vi "4080_Comms.vi"(4 "Value to display":dbl min=0.0 max=9999.9 format="%.1f", 5 "Function":T2, 6 "Channel Name":string, 9 "Address":T1) -> (1 "Reading":dbl, 2 "millisecond timer value":u32, 3 "Comment":string)   [LabVIEW 2018]
uses:
  ADAM Client/Sub VIs/ADAM Controls/Function_ADAM.ctl
  ADAM Client/Sub VIs/ADAM Controls/Address.ctl
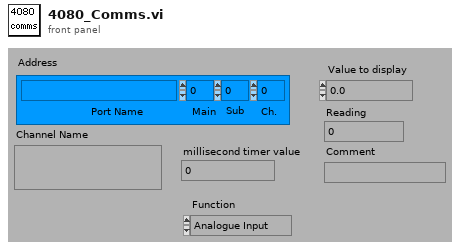
[diagram p1: front panel]
types:
  T1 = typedef "Address.ctl" = cluster{"Main":i32, "Ch.":i32, "Sub":i32, "Port Name":string}
  T2 = typedef "Function_ADAM.ctl" = enum16{"Analogue Input", "Digital Input", "Event counter", "Event rate", "Analogue Output", "Digital Output", "Relay Output"}
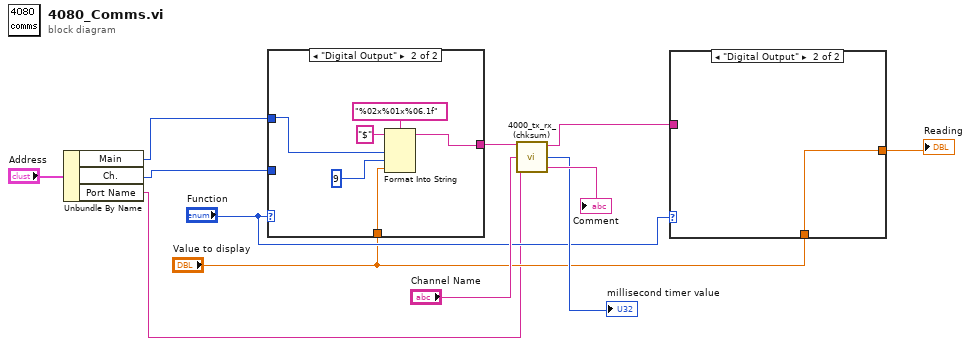
[diagram p0: block diagram]
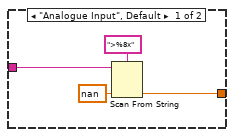
[diagram p2: hidden frame]
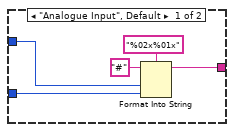
[diagram p3: hidden frame]
diagram:
  n1 = Unbundle By Name("Address") -> ("Main"=w3:i32, "Ch."=w2:i32, "Port Name"=w1:string)
  n2 = case shown="\"Digital Output\"" "Function" {
    tunnel: w2 -> [w17 _]
    tunnel: [w14 w19] -> w12
    tunnel: w3 -> [w13 w18]
    tunnel: "Value to display" -> [_ w20]
    frame "Analogue Input", Default {
      n3 = Format Into String(format string="%02x%01x", initial string="#", w13, w17) -> (resulting string=w14:string)  [unwired: 1 in, 1 out]
    }
    frame "Digital Output" {
      n4 = Format Into String(format string="%02x%01x%06.1f", initial string="$", w18, u8 9 ("Channel"), w20) -> (resulting string=w19:string)  [unwired: 1 in, 1 out]
    }
  }
  n5 = call "4000_tx_rx_(chksum).vi"("Write String"=w12, "Channel Name"="Channel Name", "Port Name"=w1) -> ("Read"=w7:string, "millisecond timer value"=→"millisecond timer value":u32, "Comment out"=→"Comment":string)  [unwired: 2 in]
  n6 = case shown="\"Digital Output\"" "Function" {
    tunnel: w7 -> [w25 _]
    tunnel: [w24 w28] -> w6
    tunnel: "Value to display" -> [_ w28]
    frame "Analogue Input", Default {
      n7 = Scan From String(format string=">%8x", input string=w25, default 1=nan ("Reading")) -> (output 1=w24:dbl)  [unwired: 2 in, 3 out]
    }
    frame "Digital Output" {
    }
  }
  "Reading" <- w6
